vi "处理信号.vi"(10 "动作":bool, 11 "空动作":bool) -> (0 "切换":bool, 3 "显示曲线":bool, 4 "判断":bool)   [LabVIEW 2018]
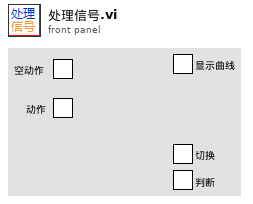
[diagram p1: front panel]
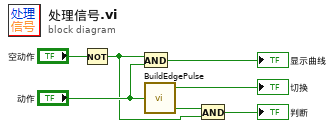
[diagram p0: block diagram]
diagram:
  n1 = Not(x="空动作") -> (.not. x?=w2:bool)
  n2 = And(x=w2, y="动作") -> (x .and. y?=→"显示曲线":bool)
  n3 = call "BuildEdgePulse.vi"("输入"="动作") -> ("下降沿"=w4:bool, "上升沿"=→"切换":bool)  [unwired: 2 in, 1 out]
  n4 = And(x=w4, y=w2) -> (x .and. y?=→"判断":bool)
